vi "Software Trigger.vi"(8 "error in (no error)":errorcluster, 11 "NI Sync in":refnum<class "NI-Sync.lvclass">) -> (0 "error out":errorcluster, 3 "NI Sync out":refnum<class "NI-Sync.lvclass">)   [LabVIEW 2025, in "Synchronization.lvlib" / "NI-Sync.lvclass"]
uses:
  NI-Sync.lvclass
  NI-Sync.lvclass/NI-Sync.ctl
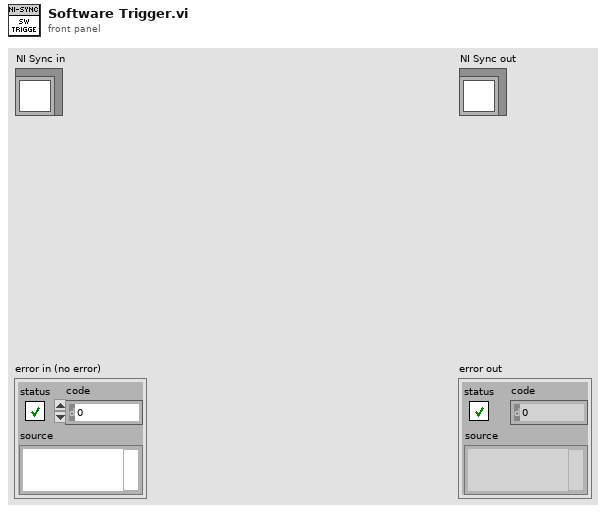
[diagram p1: front panel]
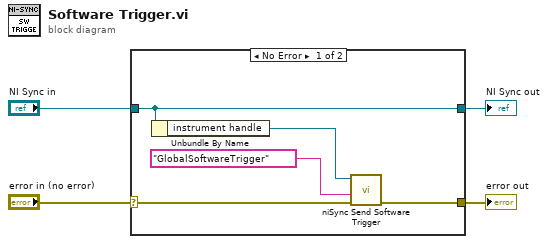
[diagram p0: block diagram]
diagram:
  n1 = case shown="No Error" "error in (no error)" {
    selector: "error in (no error)" -> [w9 w11]
    tunnel: [w8 w11] -> w3
    tunnel: [w6 w10] -> w1
    tunnel: "NI Sync in" -> [w6 w10]
    frame No Error {
      n2 = Unbundle By Name(w6) -> ("instrument handle"=w5:refnum<k15>)
      n3 = call <instrlib>:"niSync Send Software Trigger.vi"("error in (no error)"=w9, "source terminal"="GlobalSoftwareTrigger", "instrument handle"=w5) -> ("error out"=w8:errorcluster)  [unwired: 7 in, 1 out]
    }
    frame Error {
    }
  }
  "error out" <- w3
  "NI Sync out" <- w1
